vi "FTW-Message-Lossy-CreateQueue.vi"(11 "error in":errorcluster) -> (4 "Queue":refnum<queue>, 15 "error out":errorcluster)   [LabVIEW 2013, in "FTW-Message-Lossy.lvclass"]
uses:
  FTW-Message-Lossy.lvclass
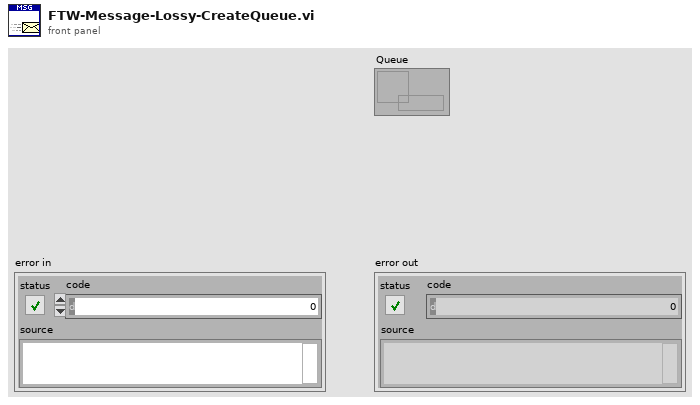
[diagram p1: front panel]
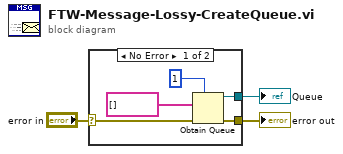
[diagram p0: block diagram]
diagram:
  n1 = case shown="No Error" "error in" {
    selector: "error in" -> [w8 w9]
    tunnel: [w7 w9] -> w2
    tunnel: [w6 _] -> w1
    frame No Error {
      n2 = Obtain Queue(max queue size (-1, unlimited)=1, element data type=string[] [] ("Parts"), error in (no error)=w8) -> (queue out=w6:refnum<queue>, error out=w7:errorcluster)  [unwired: 2 in, 1 out]
    }
    frame Error {
    }
  }
  "error out" <- w2
  "Queue" <- w1
